vi "IndexArray.vi"() -> ()   [LabVIEW 2019]
panel:
  out "subarray 2":dbl[](array[numeric])
  out "subarray":dbl[](array[numeric])
  out "element 3":dbl
  in  "2Da":dbl[][](array[numeric])=[[1.0, 2.0, 3.0, 4.0, 5.0, 6.0]]
  out "element 2":dbl
  out "element":dbl
  in  "a":dbl[](array[numeric])=[1.0, 2.0, 3.0, 4.0, 5.0, 6.0]
  # "0,0"
  # "0,1"
  # "0,2"
  # "0,3"
  # "0,4"
  # "0,5"
  # "1,0"
  # "1,1"
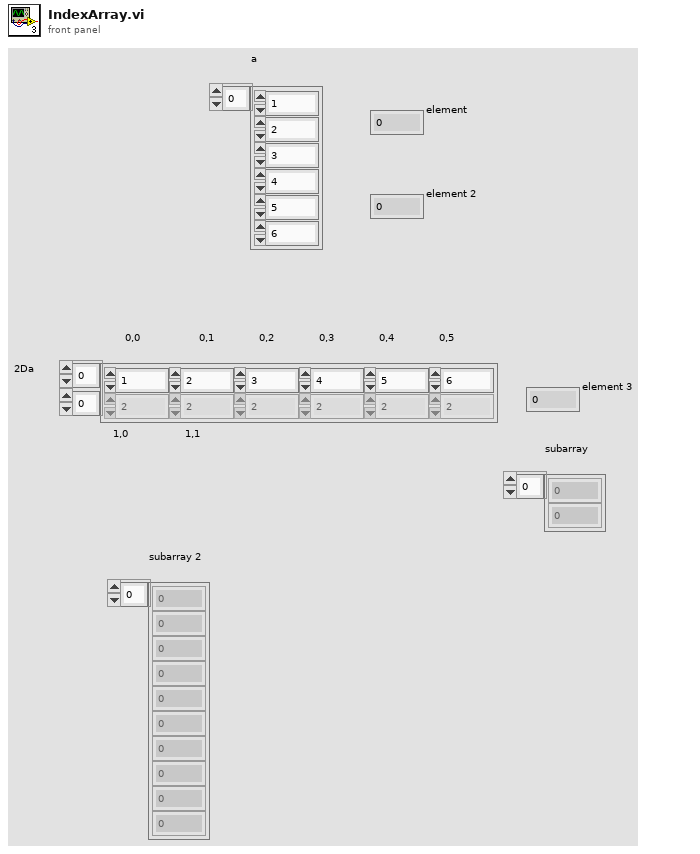
[diagram p1: front panel]
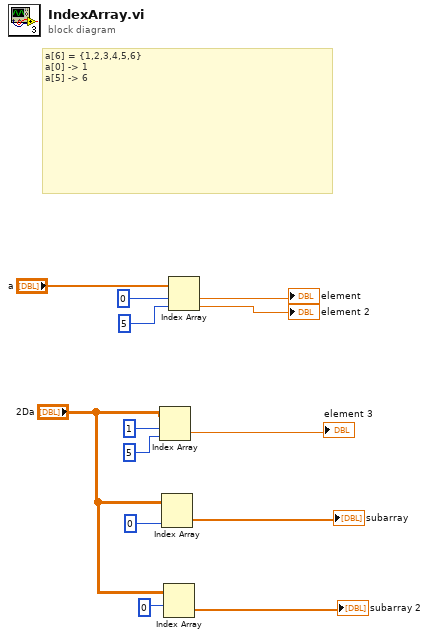
[diagram p0: block diagram]
diagram:
  # "a[6] = {1,2,3,4,5,6}\na[0] -> 1\na[5] -> 6"
  n1 = Index Array(array="2Da", index (row)=1, index (col)=5 ("index (row)")) -> (element=→"element 3":dbl)
  n2 = Index Array(array="2Da", index (col)=0 ("disabled index (col)")) -> (element=→"subarray":dbl[])  [unwired: 1 in]
  n3 = Index Array(array="2Da", index (row)=0 ("disabled index (col)")) -> (element=→"subarray 2":dbl[])  [unwired: 1 in]
  n4 = Index Array(array="a", index #1=0 ("index"), index #2=5 ("index")) -> (element #1=→"element":dbl, element #2=→"element 2":dbl)
